vi "环境温度标定.vi"(11 "环境温度信号输入":dbl) -> (3 "环境温度输出":dbl)   [LabVIEW 2016]
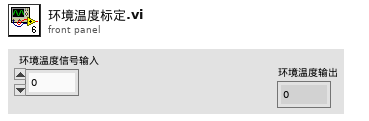
[diagram p1: front panel]
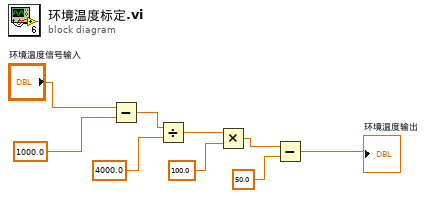
[diagram p0: block diagram]
diagram:
  n1 = Subtract(x="环境温度信号输入", y=1000.0) -> (x-y=w7:dbl)
  n2 = Divide(x=w7, y=4000.0) -> (x/y=w5:dbl)
  n3 = Multiply(x=w5, y=100.0) -> (x*y=w3:dbl)
  n4 = Subtract(x=w3, y=50.0) -> (x-y=→"环境温度输出":dbl)
